vi "ExEMCircBufROInframeSeqAdvDisp.vi"() -> ()   [LabVIEW 2010]
uses:
  CamHandle.vi
panel:
  in  "SITKFULLDISPLAYLib.SITKFullDisplay":refnum<k7>(container)
  in  "Number of images":u32=25
  in  "OK Button":bool
  out "Collecting":bool
  in  "av gain":dbl format="%.2f"
  in  "Invert Logic output":bool
  in  "Logic Output":i32
  in  "Fan":i32=1
  in  "ADC Gain":u32
  out "ADC Speed (Khz)":u32
  in  "Fast ADC":bool
  in  "X Start":u32=1 min=1 step=1
  in  "Y Bin":u32=1 min=1 step=1
  in  "X End":u32=512 min=1 max=512 step=1
  in  "X Bin":u32=1 min=1 step=1
  in  "Y Start":u32=1 min=1 step=1
  in  "Y End":u32=512 min=1 max=512 step=1
  in  "Temperature":dbl=-55.0 format="%.2f"
  in  "Exposure":dbl min=0.0 step=0.001 format="%.3f"
  out "error out":errorcluster
  in  "error in (no error)":errorcluster
  # "ExEMCircBufROInframeSeqAdvDisp:\nThis example allows a single ROI to be programmed up. It then runs in sync (nframe mode displaying  the ROI data as it comes in.\nNote: this example requires the camera support circular buffers.\nThis example also shows how to \nsetup the camera to run in over-\nlapped mode and how to set the\non-chip multiplication gain and how\nto set the readout port."
  # "Warning: you must open and run once the VI ExOpenGlobalCam.vi.\nYou only need to run it once then you can run this Example VI as many times as you want."
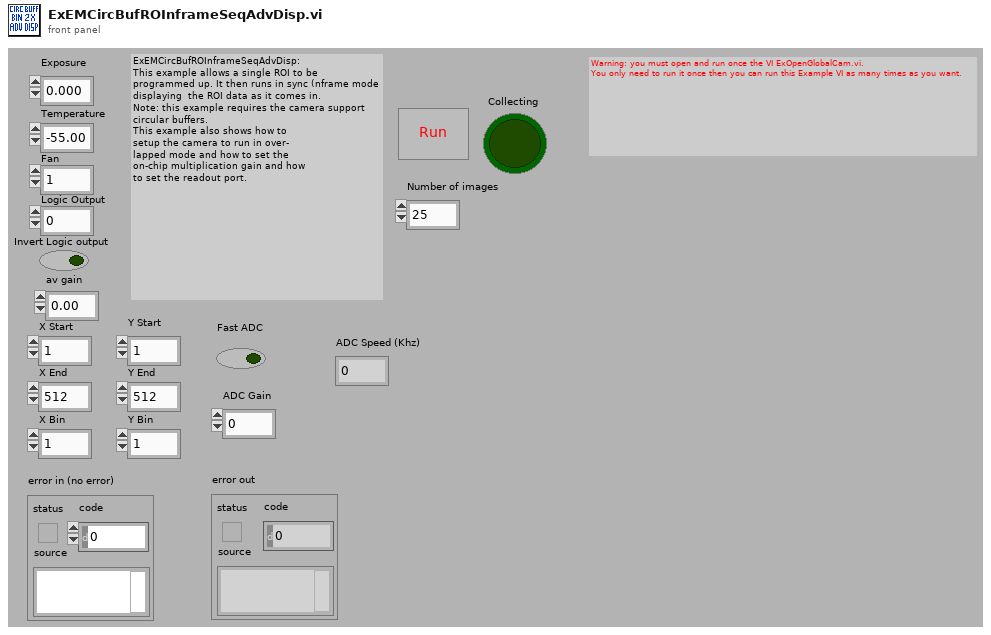
[diagram p1: front panel]
types:
  T1 = cluster{"X Start":u32, "X End":u32, "X Bin":u32, "Y Start":u32, "Y End":u32, "Y Bin":u32}
  T2 = cluster{"acquire focus mode":u32, "Exposure":dbl, "Number of images":u32, "Software accumulation":u32}
  T3 = cluster{"Camera Handle":u32, "File Handle":u32, "Image Handle":u32}
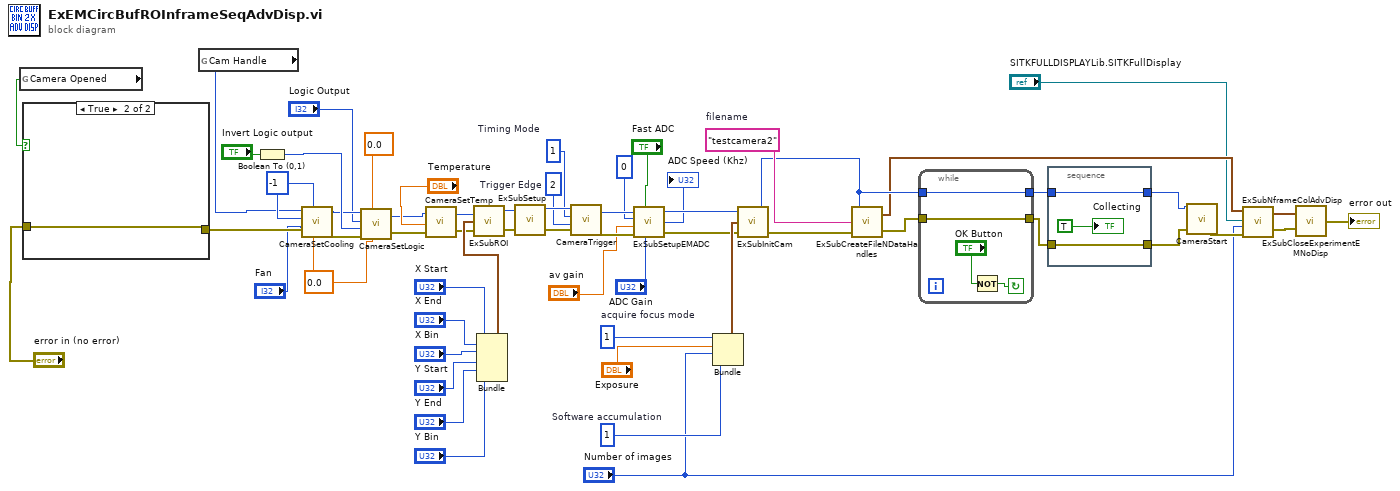
[diagram p0: block diagram]
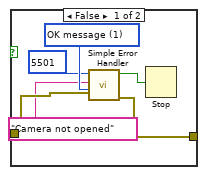
[diagram p2: hidden frame]
diagram:
  w17 = 0.0
  w18 = -1
  w50 = u32 1  # Timing Mode
  w51 = u32 2  # Trigger Edge
  w53 = u32 1  # acquire focus mode
  w52 = u32 1  # Software accumulation
  w59 = "testcamera2"  # filename
  n1 = global read "CamHandle.vi" "Camera Opened"() -> (w27:bool)
  n2 = case shown="True" w27 {
    tunnel: "error in (no error)" -> [w64 w66]
    tunnel: [w63 w66] -> w25
    frame False {
      w65 = u16 1 items=["no dialog", "OK message", "continue or stop message"] ("type of dialog (OK msg:1)")
      n3 = call <vilib>:"Simple Error Handler.vi"("error code (no error:0)"=5501, "error source (\" \")"="Camera not opened", "type of dialog (OK msg:1)"=w65, "error in (no error)"=w64) -> ("error?"=w61:bool, "error out"=w63:errorcluster)  [unwired: 1 in, 3 out]
      n4 = Stop(stop? (T)=w61) -> ()
    }
    frame True {
    }
  }
  n5 = global read "CamHandle.vi" "Cam Handle"() -> (w13:u32)
  n6 = Boolean To (0,1)(Boolean="Invert Logic output") -> (0, 1=w21:i16)
  n7 = call <userlib>:"CameraSetCooling.vi"("Reserved"=w17, "Cooling Mode"=w18, "error in (no error)"=w25, "Fan"="Fan", "Cooling"=w18, "Camera Handle"=w13) -> ("error out"=w24:errorcluster, "Camera Handle"=w20:u32)
  n8 = call <userlib>:"CameraSetLogic.vi"("Reserved 2"=w17, "Reserved"=0.0, "error in (no error)"=w24, "Invert Logic"=w21, "Logic Output"="Logic Output", "Camera Handle"=w20) -> ("error out"=w23:errorcluster, "Camera Handle"=w16:u32)
  n9 = call <userlib>:"CameraSetTemp.vi"("error in (no error)"=w23, "Temperature"="Temperature", "Camera Handle"=w16) -> ("error out"=w41:errorcluster, "Camera Handle"=w40:u32)
  n10 = Bundle("X Start"="X Start", "X End"="X End", "X Bin"="X Bin", "Y Start"="Y Start", "Y End"="Y End", "Y Bin"="Y Bin") -> (w43:T1)  [unwired: 1 in]
  n11 = call "ExSubROI.vi"("error in (no error)"=w41, "ROI"=w43, "Camera Handle"=w40) -> ("error out"=w38:errorcluster, "Camera Handle"=w42:u32)
  n12 = call "ExSubSetup.vi"("error in (no error)"=w38, "Camera Handle"=w42) -> ("error out"=w37:errorcluster, "Camera Handle"=w54:u32)
  n13 = call <userlib>:"CameraTrigger.vi"("error in"=w37, "Trigger Edge"=w51, "Timing Mode"=w50, "Camera Handle"=w54) -> ("error out"=w35:errorcluster, "Camera Handle"=w36:u32)
  n14 = call "ExSubSetupEMADC.vi"("Camera Handle"=w36, "Fast ADC"="Fast ADC", "ReadOut Port"=0, "Avalanche Gain\nOnly valid for \nport 0"="av gain", "ADC Gain"="ADC Gain", "error in (no error)"=w35) -> ("Camera Handle"=w33:u32, "ADC Speed (Khz)"=→"ADC Speed (Khz)":u32, "error out"=w34:errorcluster)
  n15 = Bundle("acquire focus mode"=w53, "Exposure"="Exposure", "Number of images"="Number of images", "Software accumulation"=w52) -> (w57:T2)  [unwired: 1 in]
  n16 = call "ExSubInitCam.vi"("error in (no error)"=w34, "Camera Information"=w57, "Camera Handle"=w33) -> ("error out"=w56:errorcluster, "Camera Handle"=w10:u32)
  n17 = call "ExSubCreateFileNDataHandles.vi"("error in (no error)"=w56, "File and Display Name"=w59, "Camera Handle"=w10) -> ("error out"=w7:errorcluster, "Handles Out"=w4:T3)
  n18 = while {
    tunnel: w10 -> [w68]
    tunnel: [w68] -> w9
    tunnel: w7 -> [w67]
    tunnel: [w67] -> w6
    stop <- w70 continue-if-true
    n19 = Not(x="OK Button") -> (.not. x?=w70:bool)
  }
  n20 = stacked-sequence {
    tunnel: w9 -> [w72]
    tunnel: [w72] -> w8
    tunnel: w6 -> [w71]
    tunnel: [w71] -> w5
    frame #0 {
      "Collecting" <- TRUE
    }
  }
  n21 = call <userlib>:"CameraStart.vi"("error in"=w5, "Camera Handle"=w8) -> ("error out"=w3:errorcluster)  [unwired: 1 out]
  n22 = call "ExSubNframeColAdvDisp.vi"("Handle Cluster"=w4, "SITKFULLDISPLAYLib.SITKFullDisplay"="SITKFULLDISPLAYLib.SITKFullDisplay", "Number of Images"="Number of images", "error in (no error)"=w3) -> ("Handle Cluster"=w11:T3, "error out"=w12:errorcluster)
  n23 = call "ExSubCloseExperimentEMNoDisp.vi"("error in (no error)"=w12, "Handles In"=w11) -> ("error out"=→"error out":errorcluster)
